vi "IDS_Disconnect.vi"(8 "error in (no error)":errorcluster, 11 "deviceHandle":i32) -> (0 "error out":errorcluster)   [LabVIEW 2016]
doc: "int IDS_DLL IDS_Disconnect();"
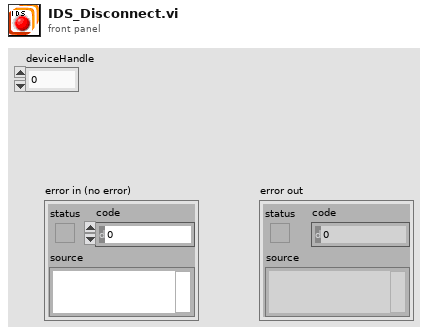
[diagram p1: front panel]
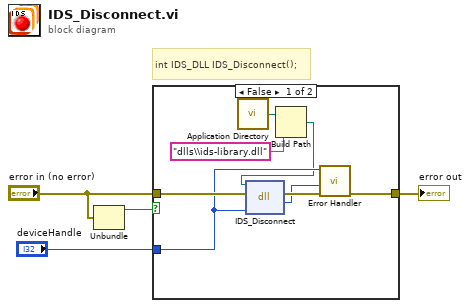
[diagram p0: block diagram]
diagram:
  # "int IDS_DLL IDS_Disconnect();"
  n1 = Unbundle("error in (no error)") -> ("status"=w1:bool)  [unwired: 2 out]
  n2 = case shown="False" w1 {
    tunnel: "error in (no error)" -> [w12 w13]
    tunnel: [w10 w13] -> w4
    tunnel: "deviceHandle" -> [w8 _]
    frame False {
      n3 = call <vilib>:"Application Directory.vi"() -> ("Application Directory"=w7:path)
      n4 = Build Path(base path=w7, name or relative path="dlls\\ids-library.dll" ("ipAddress")) -> (appended path=w5:path)
      n5 = dll-call lib="C:/Users/matheus/Desktop/LabVIEW_Draft_V1.6.0/dlls/ids-library.dll" fn="IDS_Disconnect"(path in=w5, error in=w12, "deviceHandle"=w8) -> (error out=w11:errorcluster, "return type"=w9:i32)  [unwired: 2 in, 1 out]
      n6 = call "Error Handler.vi"("error in (no error)"=w11, "error code"=w9, "deviceHandle"=w8) -> ("error out"=w10:errorcluster)  [unwired: 7 in, 1 out]
    }
    frame True {
    }
  }
  "error out" <- w4
